vi "Configure serial bus.vi"(8 "Error In":errorcluster, 11 "VISA resource name":refnum<visa-resource-name>) -> (0 "Error Out":errorcluster, 2 "Add instrument":bool, 3 "VISA resource name 2":refnum<visa-resource-name>)   [LabVIEW 2015]
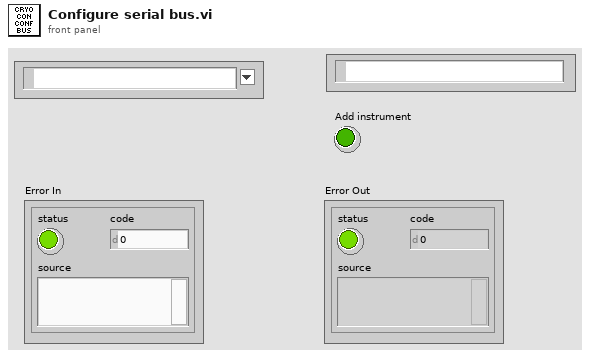
[diagram p1: front panel]
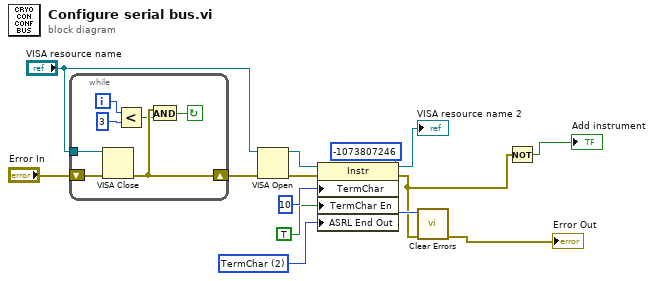
[diagram p0: block diagram]
diagram:
  w11 = u16 2 items=["None", "Last Bit", "TermChar", "Break"] ("Serial Settings:End Mode for Writes")
  n1 = while {
    tunnel: "VISA resource name" -> [w20]
    shift-right: [w16] -> w8
    shift-left: "Error In" -> [w19]
    i -> [w18]
    stop <- w15 continue-if-true
    n2 = VISA Close(VISA resource name=w20, error in (no error)=w19) -> (error out=w16:errorcluster)
    n3 = Less?(x=w18, y=3) -> (x < y?=w14:bool)
    n4 = And(x=w16, y=w14) -> (x .and. y?=w15:bool)
  }
  n5 = VISA Open(error in (no error)=w8, VISA resource name="VISA resource name") -> (VISA resource name=w6:refnum<visa-resource-name>, error out=w5:errorcluster)  [unwired: 3 in]
  n6 = property class="Instr"(reference=w6, error in=w5, "TermChar"=u8 10 ("Message Based Settings:Termination Character"), "TermChar En"=TRUE ("Message Based Settings:Termination Character Enable"), "ASRL End Out"=w11) -> (reference out=→"VISA resource name 2":refnum<visa-resource-name>, error out=w1:errorcluster)
  n7 = call <vilib>:"Clear Errors.vi"("error in (no error)"=w1, "specific error code to clear (0: all)"=-1073807246) -> ("error out"=→"Error Out":errorcluster)  [unwired: 4 in, 1 out]
  n8 = Not(x=w1) -> (.not. x?=→"Add instrument":bool)
